vi "ReadOpenMVImage.vi"(8 "error in":errorcluster, 11 "Python":T2={"session"=refnum, "PyPath"=path "/Users/crogers/GitHub/ME35_21/PythonIDE/_LVsubs/Serial/RogersSerial.py", "Processor"=enum."OpenMV", "Port"="", "version"=""}) -> (0 "error out":errorcluster, 1 "Good?":bool, 2 "size()":u32[](array[numeric])=[0, 221655862, 825503242], 3 "Python":T2={"session"=refnum, "PyPath"=path "/Users/crogers/GitHub/ME35_21/PythonIDE/_LVsubs/Serial/RogersSerial.py", "Processor"=enum."OpenMV", "Port"="", "version"=""}, 4 "image data":T1, 5 "new picture":picture)   [LabVIEW 2022 SP3]
uses:
  PythonCtrl.ctl
  Processors.ctl
  <vilib>/picture/picture.llb/imagedata.ctl
panel:
  out "VGA one":string
  out "success":string
  out "Failed":string
  out "read buffer":string
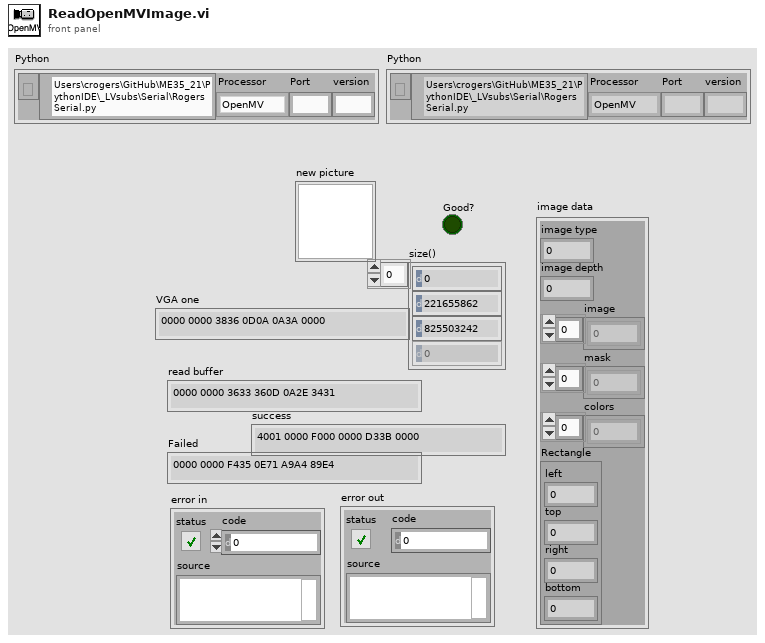
[diagram p1: front panel]
types:
  T1 = typedef "imagedata.ctl" = cluster{"image type":i32, "image depth":i32, "image":u8[], "mask":u8[], "colors":u32[], "Rectangle":cluster{"left":i16, "top":i16, "right":i16, "bottom":i16}}
  T2 = typedef "PythonCtrl.ctl" = cluster{"session":refnum<k35>, "PyPath":path, "Processor":T3, "Port":string, "version":string}
  T3 = typedef "Processors.ctl" = enum16{"SPIKE", "Pi", "Pi_ssh", "OpenMV", "Dunio"}
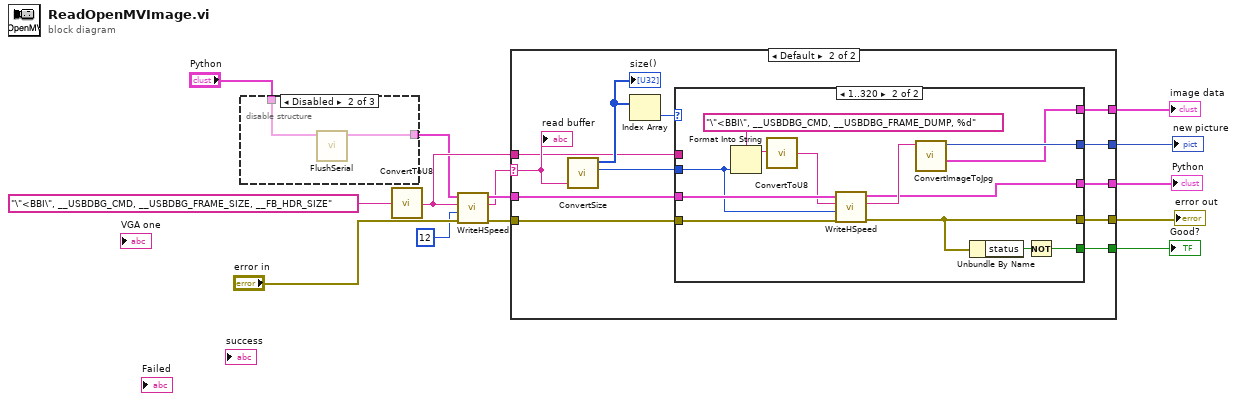
[diagram p0: block diagram]
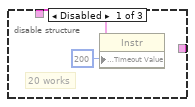
[diagram p2: hidden frame]
diagram:
  n1 = disable-structure shown="Disabled" {
    disable-tunnel: "Python" -> [w15 w18 w19]
    disable-tunnel: [_ w17 w19] -> w1
    frame Disabled {
      # "20 works"
      n2 = property class="Instr"(reference=w15, "General Settings:Timeout Value"=u32 200) -> ()  [unwired: 1 in, 2 out]
    }
    frame Disabled {
      n3 = call "FlushSerial.vi"("Python"=w18) -> ("Python"=w17:T2)  [unwired: 9 in, 1 out]
    }
    frame Enabled {
    }
  }
  n4 = call "ConvertToU8.vi"("struct"="\"<BBI\", __USBDBG_CMD, __USBDBG_FRAME_SIZE, __FB_HDR_SIZE" ("write buffer")) -> ("Binary"=w3:string)
  n5 = call "WriteHSpeed.vi"("error in"="error in", "Reply length"=12, "write buffer"=w3, "Python"=w1) -> ("error out"=w6:errorcluster, "read buffer"=w5:string, "Python"=w7:T2)  [unwired: 5 in]
  n6 = case shown="Default" w5 {
    selector: w5 -> [_ w26]
    tunnel: [w21 w33] -> w14
    tunnel: [w20 w32] -> w8
    tunnel: w7 -> [w21 w24]
    tunnel: w6 -> [w20 w30]
    tunnel: [_ w29] -> w12
    tunnel: [_ w28] -> w11
    tunnel: [_ w27] -> w10
    tunnel: w3 -> [_ w23]
    frame "" {
    }
    frame Default {
      n7 = call "ConvertSize.vi"("read buffer"=w26) -> ("# bytes"=w31:u32, "size()"=w25:u32[])  [unwired: 9 in]
      "size()" <- w25
      n8 = Index Array(array=w25) -> (element=w22:u32)  [unwired: 1 in]
      n9 = case shown="1..320" w22 {
        tunnel: [w34 w46] -> w33
        tunnel: [w35 w38] -> w32
        tunnel: w31 -> [_ w44]
        tunnel: w24 -> [w34 w47]
        tunnel: w30 -> [w35 w45]
        tunnel: [_ w40] -> w29
        tunnel: [_ w39] -> w28
        tunnel: [_ w36] -> w27
        tunnel: w23 -> [_ _]
        frame Default {
        }
        frame 1..320 {
          n10 = Format Into String(format string="\"<BBI\", __USBDBG_CMD, __USBDBG_FRAME_DUMP, %d" ("write buffer"), w44) -> (resulting string=w42:string)  [unwired: 2 in, 1 out]
          n11 = call "ConvertToU8.vi"("struct"=w42) -> ("Binary"=w41:string)
          n12 = call "WriteHSpeed.vi"("error in"=w45, "Reply length"=w44, "write buffer"=w41, "Python"=w47) -> ("error out"=w38:errorcluster, "read buffer"=w48:string, "Python"=w46:T2)  [unwired: 5 in]
          n13 = call "ConvertImageToJpg.vi"("buffer"=w48) -> ("image data"=w39:T1, "new picture"=w40:picture)  [unwired: 9 in]
          n14 = Unbundle By Name(w38) -> ("status"=w37:bool)
          n15 = Not(x=w37) -> (.not. x?=w36:bool)
        }
      }
      "read buffer" <- w26
    }
  }
  "Python" <- w14
  "error out" <- w8
  "new picture" <- w12
  "image data" <- w11
  "Good?" <- w10
